vi "3.4.vi"() -> ()   [LabVIEW 2017]
panel:
  out "长度":i32
  out "字符串 3":string
  in  "字符串 2":string
  in  "数值":dbl
  in  "字符串":string
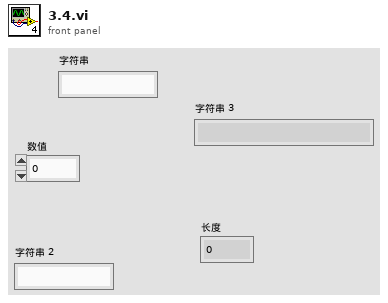
[diagram p1: front panel]
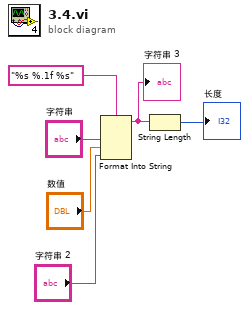
[diagram p0: block diagram]
diagram:
  n1 = Format Into String(format string="%s %.1f %s" ("格式字符串"), "字符串", "数值", "字符串 2") -> (resulting string=w3:string)  [unwired: 2 in, 1 out]
  "字符串 3" <- w3
  n2 = String Length(string=w3) -> (length=→"长度":i32)
